vi "Adjusted Palette Range.vi"(9 "Image Min":sgl, 11 "Image Max":sgl) -> (1 "Palette Range Min":sgl, 2 "delta":sgl, 3 "Palette Range Max":sgl)   [LabVIEW 2021, in "Image.lvlib"]
uses:
  Image.lvlib
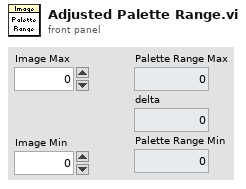
[diagram p1: front panel]
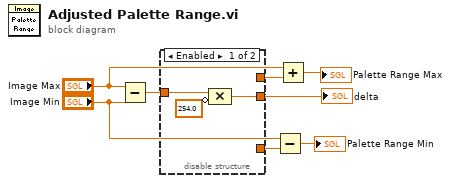
[diagram p0: block diagram]
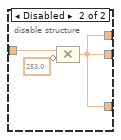
[diagram p2: hidden frame]
diagram:
  n1 = Subtract(x="Image Max", y="Image Min") -> (x-y=w8:sgl)
  n2 = disable-structure shown="Enabled" {
    disable-tunnel: w8 -> [w11 w14]
    disable-tunnel: [_ w12] -> w2
    disable-tunnel: [_ w12] -> w1
    disable-tunnel: [w9 w12] -> w3
    frame Enabled {
      n3 = Compound Arithmetic op=MULTIPLY(w11, invert sgl 254.0 ("value")) -> (w9:sgl)
    }
    frame Disabled {
      n4 = Compound Arithmetic op=MULTIPLY(w14, invert sgl 253.0 ("value")) -> (w12:sgl)
    }
  }
  "delta" <- w3
  n5 = Subtract(x="Image Min", y=w1) -> (x-y=→"Palette Range Min":sgl)
  n6 = Add(x="Image Max", y=w2) -> (x+y=→"Palette Range Max":sgl)
